vi "Write summaryState.vi"(10 "ComponentState.lvclass":refnum<class "ComponentState.lvclass">, 11 "ComponentData in":refnum<class "ComponentData.lvclass">) -> (3 "ComponentData out":refnum<class "ComponentData.lvclass">)   [LabVIEW 2013, in "ComponentData.lvlib" / "ComponentData.lvclass"]
uses:
  <userlib>/Common/Component/Application/RT/ComponentData/ComponentData/ComponentData.lvclass
  <userlib>/Common/Component/Application/RT/ComponentData/ComponentState/ComponentState/ComponentState.lvclass
  <userlib>/Common/Component/Application/RT/ComponentData/ComponentData/ComponentData.lvclass/ComponentData.ctl
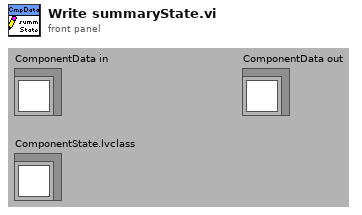
[diagram p1: front panel]
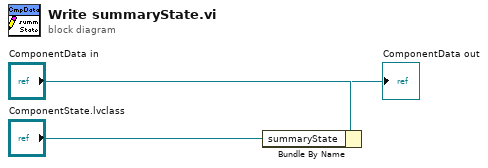
[diagram p0: block diagram]
diagram:
  n1 = Bundle By Name(cluster="ComponentData in", "summaryState"="ComponentState.lvclass") -> (→"ComponentData out":refnum<class "ComponentData.lvclass">)
